vi "Multiple Registration - Right.vi"() -> ()   [LabVIEW 2011]
panel:
  out "Time Process 3 was Stopped":timestamp
  out "Process 3":timestamp
  out "Time Process 2 was Stopped":timestamp
  out "Process 2":timestamp
  out "Time Process 1 was Stopped":timestamp
  in  "stop":bool
  out "Process 1":timestamp
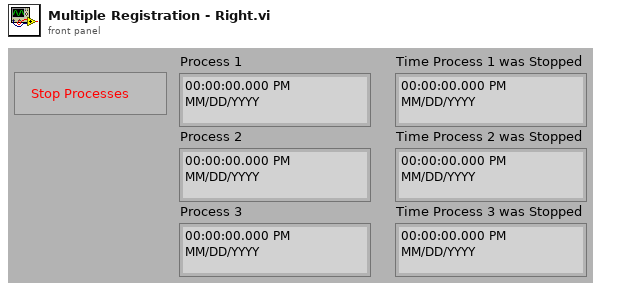
[diagram p1: front panel]
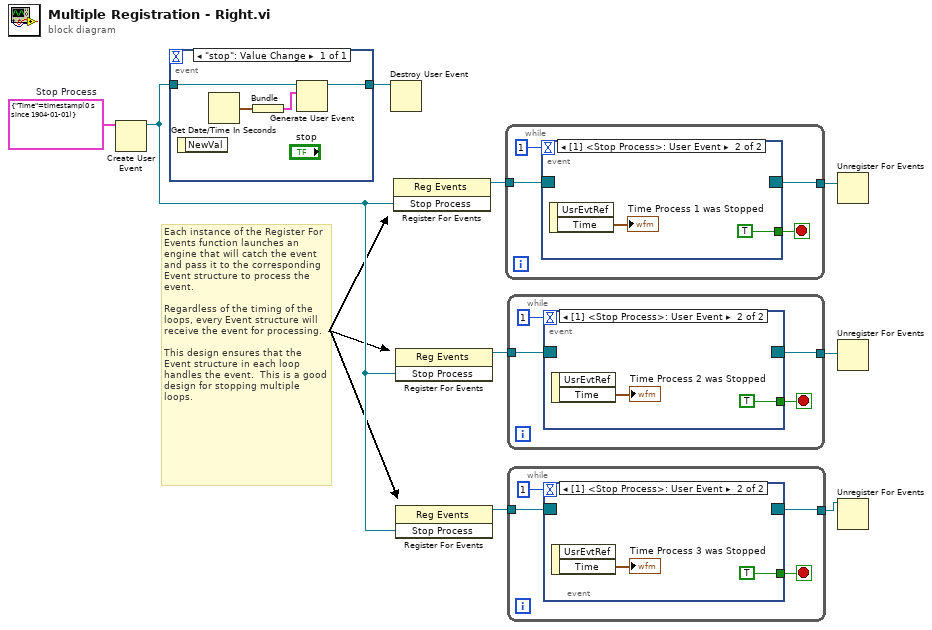
[diagram p0: block diagram]
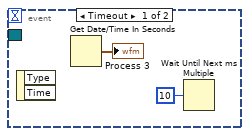
[diagram p2: hidden frame]
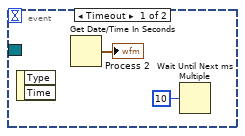
[diagram p3: hidden frame]
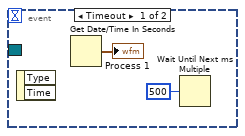
[diagram p4: hidden frame]
diagram:
  w9 = cluster{"Time":timestamp} {"Time"=timestamp(0 s since 1904-01-01)}  # Stop Process
  # "Each instance of the Register For Events function launches an engine that will catch the event and pass it to the corresponding  Event structure to process the event.\n\nRegardless of the timing of the loops, every Event structure will receive the event for processing.\n\nThis design ensures that the Event structure in each loop handles the event.  This is a good design for stopping multiple loops."
  n1 = Create User Event(user event datatype=w9) -> (user event=w8:refnum<user-event>)  [unwired: 1 in, 1 out]
  n2 = event shown="[0] \"stop\": Value Change" {
    selector: _ -> [_]
    dyn-events: _ -> [_]
    timeout: _ -> [_]
    tunnel: w8 -> [w13]
    tunnel: [w10] -> w7
    event "stop": Value Change {
      n3 = event-data() -> ()  [unwired: 1 in, 1 out]
      n4 = Get Date/Time In Seconds() -> (seconds since 1Jan1904=w12:timestamp)
      n5 = Bundle("seconds since 1Jan1904"=w12) -> (w11:cluster{"seconds since 1Jan1904":timestamp})  [unwired: 1 in]
      n6 = Generate User Event(user event=w13, event data cluster=w11) -> (user event out=w10:refnum<user-event>)  [unwired: 1 in, 1 out]
    }
  }
  n7 = Destroy User Event(user event=w7) -> ()  [unwired: 1 in, 1 out]
  n8 = register-events(w8) -> (reference out=w6:refnum<event-registration>)  [unwired: 2 in, 1 out]
  n9 = register-events(w8) -> (reference out=w5:refnum<event-registration>)  [unwired: 2 in, 1 out]
  n10 = register-events(w8) -> (reference out=w4:refnum<event-registration>)  [unwired: 2 in, 1 out]
  n11 = while {
    tunnel: w6 -> [w16]
    tunnel: [w14] -> w3
    stop <- w15 stop-if-true
    n12 = event shown="[1] <Stop Process>: User Event" {
      selector: w16 -> [_ _]
      dyn-events: [_ _] -> w14
      timeout: 1 -> [_ _]
      tunnel: [_ TRUE] -> w15
      event Timeout {
        n13 = event-data() -> ()  [unwired: 1 in, 2 out]
        n14 = Get Date/Time In Seconds() -> (seconds since 1Jan1904=→"Process 1":timestamp)
        n15 = Wait Until Next ms Multiple(millisecond multiple=u32 500) -> ()  [unwired: 1 out]
      }
      event User Event {
        n16 = event-data() -> ("Time"=→"Time Process 1 was Stopped":timestamp)  [unwired: 1 in, 1 out]
      }
    }
  }
  n17 = while {
    tunnel: w5 -> [w24]
    tunnel: [w22] -> w2
    stop <- w23 stop-if-true
    n18 = event shown="[1] <Stop Process>: User Event" {
      selector: w24 -> [_ _]
      dyn-events: [_ _] -> w22
      timeout: 1 -> [_ _]
      tunnel: [_ TRUE] -> w23
      event Timeout {
        n19 = event-data() -> ()  [unwired: 1 in, 2 out]
        n20 = Get Date/Time In Seconds() -> (seconds since 1Jan1904=→"Process 2":timestamp)
        n21 = Wait Until Next ms Multiple(millisecond multiple=u32 10) -> ()  [unwired: 1 out]
      }
      event User Event {
        n22 = event-data() -> ("Time"=→"Time Process 2 was Stopped":timestamp)  [unwired: 1 in, 1 out]
      }
    }
  }
  n23 = while {
    tunnel: w4 -> [w32]
    tunnel: [w30] -> w1
    stop <- w31 stop-if-true
    n24 = event shown="[1] <Stop Process>: User Event" {
      selector: w32 -> [_ _]
      dyn-events: [_ _] -> w30
      timeout: 1 -> [_ _]
      tunnel: [_ TRUE] -> w31
      event Timeout {
        n25 = event-data() -> ()  [unwired: 1 in, 2 out]
        n26 = Get Date/Time In Seconds() -> (seconds since 1Jan1904=→"Process 3":timestamp)
        n27 = Wait Until Next ms Multiple(millisecond multiple=u32 10) -> ()  [unwired: 1 out]
      }
      event User Event {
        n28 = event-data() -> ("Time"=→"Time Process 3 was Stopped":timestamp)  [unwired: 1 in, 1 out]
      }
    }
  }
  n29 = Unregister For Events(event registration refnum=w3) -> ()  [unwired: 1 in, 1 out]
  n30 = Unregister For Events(event registration refnum=w2) -> ()  [unwired: 1 in, 1 out]
  n31 = Unregister For Events(event registration refnum=w1) -> ()  [unwired: 1 in, 1 out]
